vi "WFGConfigureSingleCh.vi"(0 "object in":refnum<class "AD2_WFG_SDK.lvclass">, 2 "Ch":T1={"idxChannel"=0, "Settings out of range"=FALSE, "Carrier"={"Frequency (Hz)"=1000.0, "Amplitude (V)"=1.0, "Offset(V)"=0.0, "Symmetry(%) "=50.0, "Phase(Deg)"=0.0, "Function"=1, "Enable"=FALSE}, "Trigger"={"secRun(0=Cont)"=0.0, "secWait"=0.0, "cRepeat(0=inf)"=0, "Repeat Trigger"=FALSE, "TrigrSrc"=enum."trigrsrcNone"}, "FM Mod"={"Frequency (Hz)"=1000.0, "Amplitude (%)"=1.0, "Offset(V)"=0.0, "Symmetry(%) "=50.0, "Phase(Deg)"=0.0, "Function 2"=1, "Enable"=FALSE}} {"FM Mod"."Function 2" items=["DC"=0, "Sine"=1, "Square"=2, "Triangle"=3, "RampUp"=4, "RampDown"=5, "Noise"=6, "Pulse"=7, "Custom"=30]; "Carrier"."Function" items=["DC"=0, "Sine"=1, "Square"=2, "Triangle"=3, "RampUp"=4, "RampDown"=5, "Noise"=6, "Pulse"=7, "Custom"=30]}, 5 "error in (no error)":errorcluster) -> (14 "object out":refnum<class "AD2_WFG_SDK.lvclass">, 16 "Ch out":T1={"idxChannel"=0, "Settings out of range"=FALSE, "Carrier"={"Frequency (Hz)"=1000.0, "Amplitude (V)"=1.0, "Offset(V)"=0.0, "Symmetry(%) "=50.0, "Phase(Deg)"=0.0, "Function"=1, "Enable"=FALSE}, "Trigger"={"secRun(0=Cont)"=0.0, "secWait"=0.0, "cRepeat(0=inf)"=0, "Repeat Trigger"=FALSE, "TrigrSrc"=enum."trigrsrcNone"}, "FM Mod"={"Frequency (Hz)"=1000.0, "Amplitude (%)"=1.0, "Offset(V)"=0.0, "Symmetry(%) "=50.0, "Phase(Deg)"=0.0, "Function 2"=1, "Enable"=FALSE}} {"FM Mod"."Function 2" items=["DC"=0, "Sine"=1, "Square"=2, "Triangle"=3, "RampUp"=4, "RampDown"=5, "Noise"=6, "Pulse"=7, "Custom"=30]; "Carrier"."Function" items=["DC"=0, "Sine"=1, "Square"=2, "Triangle"=3, "RampUp"=4, "RampDown"=5, "Noise"=6, "Pulse"=7, "Custom"=30]}, 19 "error out":errorcluster)   [LabVIEW 2021, in "AD2_WFG_SDK.lvclass"]
uses:
  AD2_WFG_SDK.lvclass
  WFGCh.ctl
  AD2TriggerSources.ctl
  AD2_SDK_class/AD2_SDK.lvclass
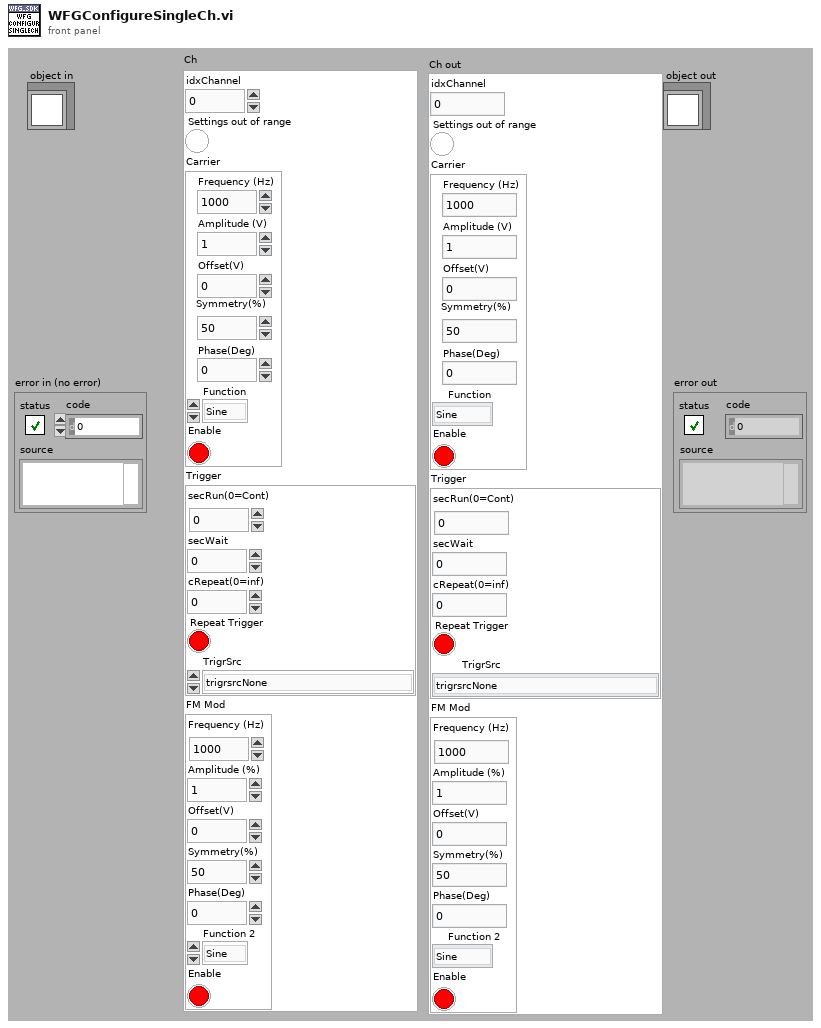
[diagram p1: front panel]
types:
  T1 = typedef "AD2_WFG_SDK.lvclass/WFGCh.ctl" = cluster{"idxChannel":i32, "Settings out of range":bool, "Carrier":cluster{"Frequency (Hz)":dbl, "Amplitude (V)":dbl, "Offset(V)":dbl, "Symmetry(%) ":dbl, "Phase(Deg)":dbl, "Function":u16, "Enable":bool}, "Trigger":cluster{"secRun(0=Cont)":dbl, "secWait":dbl, "cRepeat(0=inf)":i32, "Repeat Trigger":bool, "TrigrSrc":T2}, "FM Mod":cluster{"Frequency (Hz)":dbl, "Amplitude (%)":dbl, "Offset(V)":dbl, "Symmetry(%) ":dbl, "Phase(Deg)":dbl, "Function 2":u16, "Enable":bool}}
  T2 = typedef "AD2_SDK.lvclass/AD2TriggerSources.ctl" = enum8{"trigrsrcNone", "trigsrcPC", "trigsrcDetectorAnalogIn", "trigsrcDetectorDigitalIn", "trigsrcAnalogIn", "trigsrcDigitalIn", "trigsrcDigitalOut", "trigsrcAnalogOut1", "trigsrcAnalogOut2", "trigsrcAnalogOut3", "trigsrcAnalogOut4", "trigsrcExternal1", "trigsrcExternal2", "trigsrcExternal3", "trigsrcExternal4", ""}
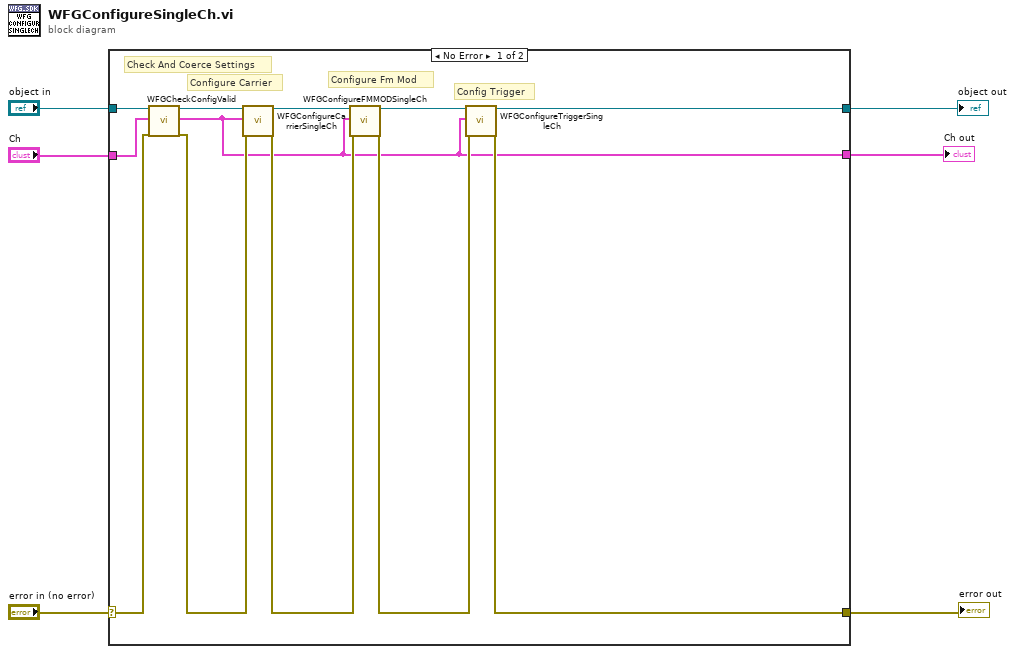
[diagram p0: block diagram]
diagram:
  n1 = case shown="No Error" "error in (no error)" {
    selector: "error in (no error)" -> [w12 w20]
    tunnel: [w10 w20] -> w5
    tunnel: [w9 w19] -> w3
    tunnel: "object in" -> [w13 w19]
    tunnel: "Ch" -> [w7 _]
    tunnel: [w8 _] -> w1
    frame No Error {
      # "Check And Coerce Settings"
      # "Configure Fm Mod"
      # "Config Trigger"
      # "Configure Carrier"
      n2 = call-dynamic "WFGCheckConfigValid.vi"("object in"=w13, "Ch"=w7, "error in (no error)"=w12) -> ("object out"=w14:refnum<class "AD2_WFG_SDK.lvclass">, "Ch Out"=w8:T1, "error out"=w11:errorcluster)  [unwired: 13 in, 1 out]
      n3 = call-dynamic "WFGConfigureCarrierSingleCh.vi"("object in"=w14, "Ch"=w8, "error in (no error)"=w11) -> ("object out"=w18:refnum<class "AD2_WFG_SDK.lvclass">, "error out"=w16:errorcluster)  [unwired: 15 in]
      n4 = call-dynamic "WFGConfigureFMMODSingleCh.vi"("object in"=w18, "Ch"=w8, "error in (no error)"=w16) -> ("object out"=w17:refnum<class "AD2_WFG_SDK.lvclass">, "error out"=w15:errorcluster)  [unwired: 15 in]
      n5 = call-dynamic "WFGConfigureTriggerSingleCh.vi"("object in"=w17, "Ch"=w8, "error in (no error)"=w15) -> ("object out"=w9:refnum<class "AD2_WFG_SDK.lvclass">, "error out"=w10:errorcluster)  [unwired: 15 in]
    }
    frame Error {
    }
  }
  "error out" <- w5
  "object out" <- w3
  "Ch out" <- w1
